vi "testToolkitErrorHandlingAddCallerToApiViListIsReentrant.vi.vi"(8 "error in (no error)":errorcluster, 11 "TesCase in":refnum<class "EasyXMLTest.lvclass">) -> (0 "error out":errorcluster, 3 "TesCase out":refnum<class "EasyXMLTest.lvclass">)   [LabVIEW 2013, in "EasyXMLTest.lvclass"]
uses:
  EasyXMLTest.lvclass
  Test Support/Reentrant Setting Requirement - Enum.ctl
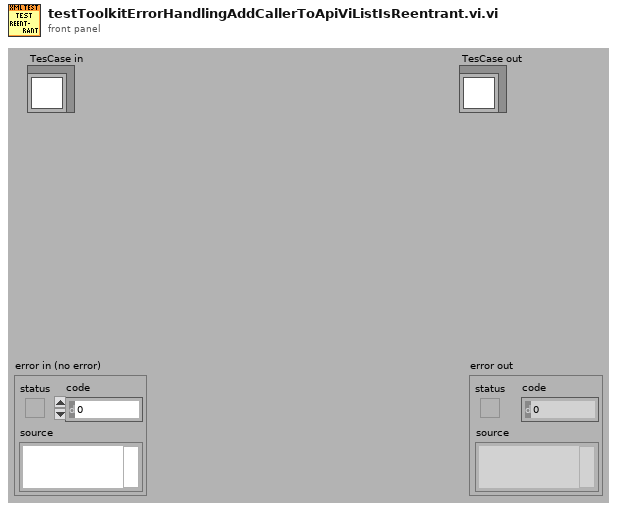
[diagram p1: front panel]
types:
  T1 = typedef "EasyXMLTest.lvclass/Reentrant Setting Requirement - Enum.ctl" = enum16{"reentrant", "non-reentrant"}
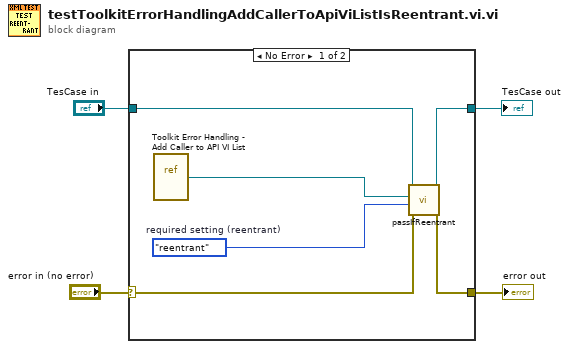
[diagram p0: block diagram]
diagram:
  n1 = case shown="No Error" "error in (no error)" {
    selector: "error in (no error)" -> [w6 w12]
    tunnel: [w7 w12] -> w3
    tunnel: [w8 w11] -> w1
    tunnel: "TesCase in" -> [w9 w11]
    frame No Error {
      w5 = Reentrant_Setting_Requirement_-_Enum."reentrant"  # required setting (reentrant)
      n2 = vi-ref "Toolkit Error Handling - Add Caller to API VI List.vi"() -> (w10:refnum<vi>)
      n3 = call "passIfReentrant.vi"("error in (no error)"=w6, "required setting (reentrant)"=w5, "VI Refnum"=w10, "TestCase in"=w9) -> ("error out"=w7:errorcluster, "TestCase out"=w8:refnum<class "EasyXMLTest.lvclass">)  [unwired: 6 in]
    }
    frame Error {
    }
  }
  "error out" <- w3
  "TesCase out" <- w1
